vi "Write angles.lvclass.vi"(8 "error in (no error)":errorcluster, 10 "angles.lvclass":refnum<class "angles.lvclass">, 11 "AG in":refnum<class "AG.lvclass">) -> (0 "error out":errorcluster, 3 "AG out":refnum<class "AG.lvclass">)   [LabVIEW 2018, in "AG.lvclass"]
uses:
  AG.lvclass
  Device/angles/angles.lvclass
  AG.lvclass/AG.ctl
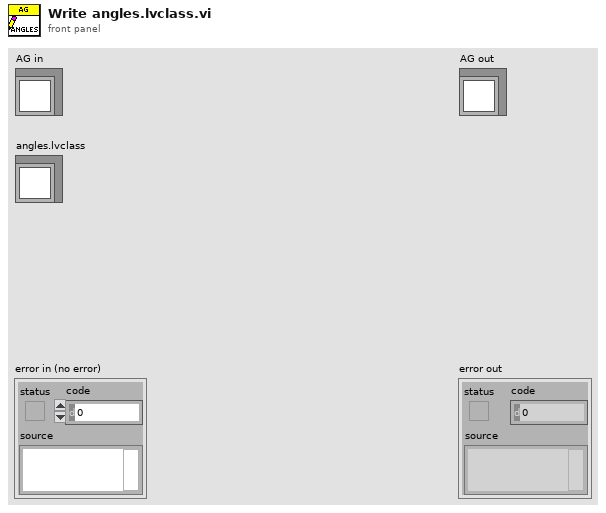
[diagram p1: front panel]
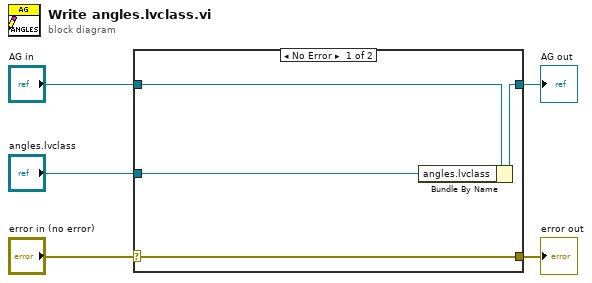
[diagram p0: block diagram]
diagram:
  n1 = case shown="No Error" "error in (no error)" {
    selector: "error in (no error)" -> [w9 w10]
    tunnel: [w9 w10] -> w4
    tunnel: [w7 w11] -> w2
    tunnel: "AG in" -> [w8 w11]
    tunnel: "angles.lvclass" -> [w6 _]
    frame No Error {
      n2 = Bundle By Name(cluster=w8, "angles.lvclass"=w6) -> (w7:refnum<class "AG.lvclass">)
    }
    frame Error {
    }
  }
  "error out" <- w4
  "AG out" <- w2
